vi "Log Events.vi"(2 "File Name":string, 3 "Log Path":path, 4 "Error In":errorcluster, 5 "Event":string, 6 "Time Format":string="%y/%m/%d; %H:%M:%S%3u", 7 "Log Command":T1) -> (0 "Error Out":errorcluster, 1 ">10MB":bool)   [LabVIEW 2018]
uses:
  Type Defs/Log Command.ctl
  <userlib>/_OpenG.lib/file/file.llb/Strip Path Extension - String__ogtk.vi
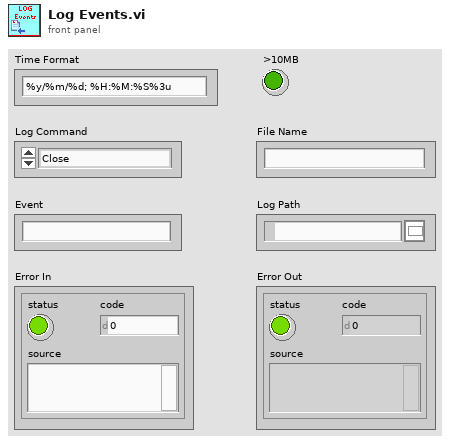
[diagram p1: front panel]
types:
  T1 = typedef "Log Command.ctl" = enum16{"Close", "Write", "Open", "No Command"}
  T2 = enum16{"open", "replace", "create", "open or create", "replace or create", "replace or create with confirmation"}
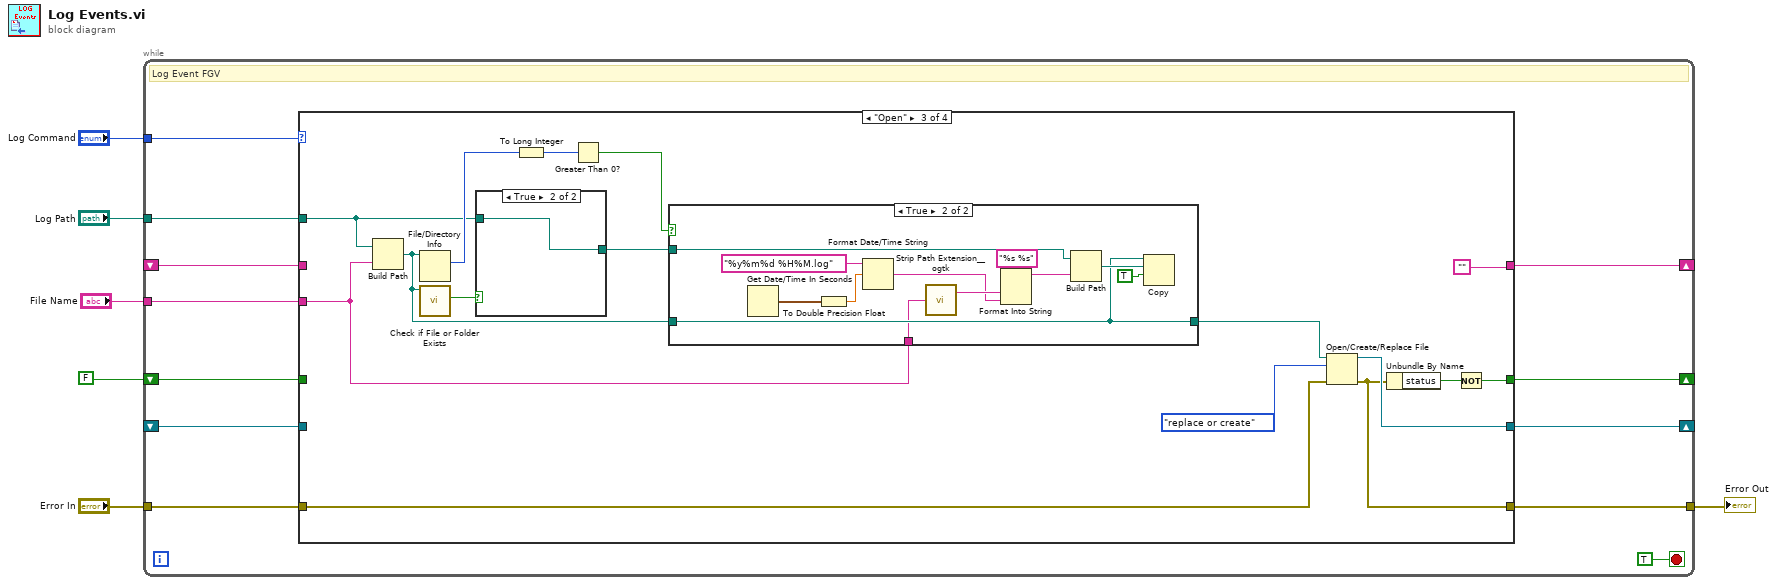
[diagram p0: block diagram]
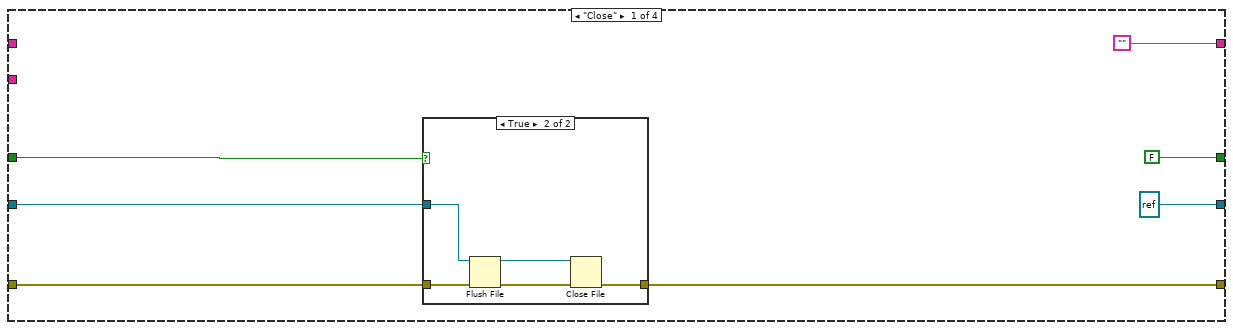
[diagram p2: hidden frame]
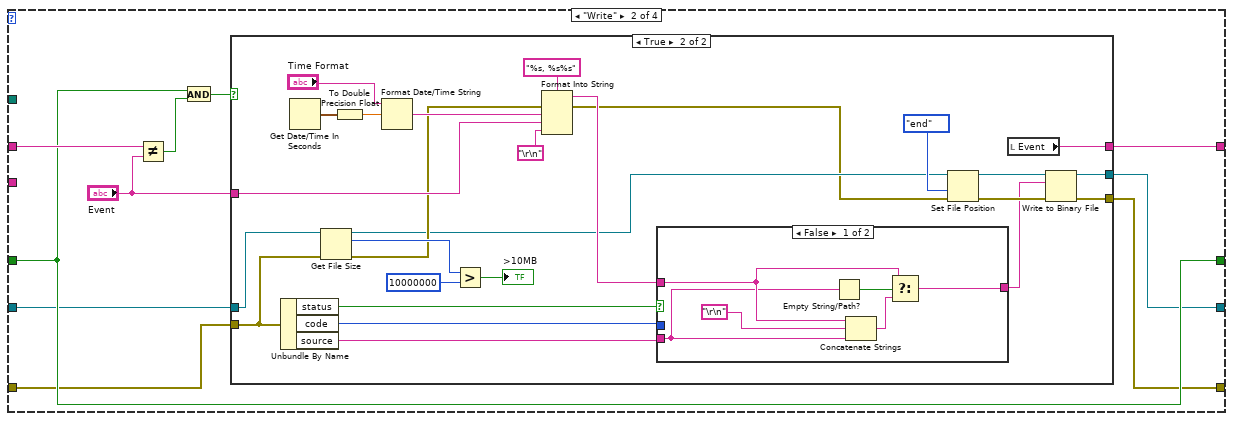
[diagram p4: hidden frame]
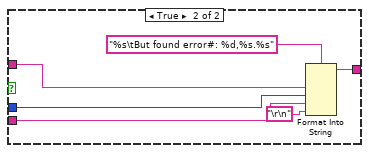
[diagram p6: hidden frame]
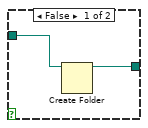
[diagram p7: hidden frame]
diagram:
  n1 = while {
    tunnel: "Error In" -> [w18]
    tunnel: [w17] -> w5
    tunnel: "Log Command" -> [w15]
    tunnel: "Log Path" -> [w14]
    tunnel: "File Name" -> [w13]
    shift-right: [w7] -> _
    shift-left: _ -> [w12]
    shift-right: [w10] -> _
    shift-left: FALSE -> [w11]
    shift-right: [w8] -> _
    shift-left: _ -> [w9]
    stop <- TRUE stop-if-true
    # "Log Event FGV"
    n2 = case shown="\"Open\"" w15 {
      tunnel: w18 -> [w24 w37 w86 w118]
      tunnel: [w22 w35 w87 w118] -> w17
      tunnel: w14 -> [_ _ w85 _]
      tunnel: w13 -> [_ _ w83 _]
      tunnel: w12 -> [w23 w34 _ w116]
      tunnel: w11 -> [w25 w39 _ w117]
      tunnel: [FALSE w39 w89 w117] -> w10
      tunnel: [refnum<file> refnum ("refnum out") w33 w88 w116] -> w7
      tunnel: w9 -> [_ w40 _ w115]
      tunnel: ["" w32 "" w115] -> w8
      frame "Close" {
        n3 = case shown="True" w25 {
          tunnel: w24 -> [w26 w28]
          tunnel: w23 -> [_ w29]
          tunnel: [w26 w27] -> w22
          frame False {
          }
          frame True {
            n4 = Flush File(refnum=w29, error in=w28) -> (refnum out=w30:refnum<file>, error out=w31:errorcluster)
            n5 = Close File(refnum=w30, error in=w31) -> (error out=w27:errorcluster)  [unwired: 1 out]
          }
        }
      }
      frame "Write" {
        n6 = Not Equal?(x=w40, y="Event") -> (x != y?=w41:bool)
        n7 = And(x=w39, y=w41) -> (x .and. y?=w38:bool)
        n8 = case shown="True" w38 {
          tunnel: w37 -> [w44 w56]
          tunnel: "Event" -> [w42 w65]
          tunnel: [w44 w49] -> w35
          tunnel: w34 -> [w43 w57]
          tunnel: [w43 w47] -> w33
          tunnel: [w42 w45] -> w32
          frame False {
          }
          frame True {
            n9 = Unbundle By Name(w56) -> ("status"=w64:bool, "code"=w63:i32, "source"=w62:string)
            n10 = Get Date/Time In Seconds() -> (seconds since 1Jan1904=w66:timestamp)
            n11 = Get File Size(file=w57, error in=w56) -> (refnum out=w50:refnum<file>, size (in bytes)=w59:i64, 0:w55:errorcluster)
            n12 = To Double Precision Float(number=w66) -> (double precision float=w70:dbl)
            n13 = Format Date/Time String(time format string (%c)="Time Format", seconds (now)=w70) -> (date/time string=w69:string)  [unwired: 1 out]
            n14 = Greater?(x=w59, y=i64 10000000) -> (0:→">10MB":bool)
            n15 = Format Into String(format string="%s, %s%s" ("Format String"), error in=w55, w69, w65, "\r\n") -> (resulting string=w61:string, error out=w48:errorcluster)  [unwired: 1 in]
            n16 = case shown="False" w64 {
              tunnel: w63 -> [_ w82]
              tunnel: w61 -> [w74 w81]
              tunnel: [w71 w79] -> w46
              tunnel: w62 -> [w72 w78]
              frame False {
                n17 = Empty String/Path?(string/path=w72) -> (empty?=w76:bool)
                n18 = Concatenate Strings(w74, "\r\n", w72) -> (w75:string)
                n19 = Select(t=w74, s=w76, f=w75) -> (s? t:f=w71:string)
              }
              frame True {
                n20 = Format Into String(format string="%s\tBut found error#: %d,%s.%s" ("Format String"), w81, w82, w78, "\r\n") -> (resulting string=w79:string)  [unwired: 2 in, 1 out]
              }
            }
            n21 = Set File Position(refnum=w50, from (0:start)=enum16{"start", "end", "current"}."end" ("pos mode (0:2)"), error in=w48) -> (refnum out=w52:refnum<file>, error out=w51:errorcluster)  [unwired: 1 out]
            n22 = local read "Event"() -> (w45:string)
            n23 = Write to Binary File(file (use dialog)=w52, data=w46, error in=w51) -> (refnum out=w47:refnum<file>, error out=w49:errorcluster)  [unwired: 1 in, 3 out]
          }
        }
      }
      frame "Open" {
        n24 = Build Path(base path=w85, name or relative path=w83) -> (appended path=w90:path)
        n25 = File/Directory Info(path=w90) -> (size=w96:i64)  [unwired: 1 in, 6 out]
        n26 = call <vilib>:"Check if File or Folder Exists.vi"("path"=w90) -> ("file or folder exists?"=w91:bool)  [unwired: 8 in, 2 out]
        n27 = case shown="True" w91 {
          tunnel: [w100 w101] -> w92
          tunnel: w85 -> [w99 w101]
          frame False {
            n28 = Create Folder(path (use dialog)=w99) -> (created path=w100:path)  [unwired: 2 in, 2 out]
          }
          frame True {
          }
        }
        n29 = To Long Integer(number=w96) -> (32bit integer=w97:i32)
        n30 = Greater Than 0?(x=w97) -> (x > 0?=w95:bool)
        n31 = case shown="True" w95 {
          tunnel: w90 -> [w102 w108]
          tunnel: w92 -> [_ w114]
          tunnel: [w102 w108] -> w94
          tunnel: w83 -> [_ w103]
          frame False {
          }
          frame True {
            n32 = Get Date/Time In Seconds() -> (seconds since 1Jan1904=w112:timestamp)
            n33 = To Double Precision Float(number=w112) -> (double precision float=w113:dbl)
            n34 = Format Date/Time String(time format string (%c)="%y%m%d %H%M.log", seconds (now)=w113) -> (date/time string=w104:string)  [unwired: 1 out]
            n35 = call-poly <userlib>:"Strip Path Extension__ogtk.vi"("path"=w103) -> ("root"=w106:string)  [unwired: 1 out]
            n36 = Format Into String(format string="%s %s", w106, w104) -> (resulting string=w105:string)  [unwired: 2 in, 1 out]
            n37 = Build Path(base path=w114, name or relative path=w105) -> (appended path=w110:path)
            n38 = Copy(9:TRUE ("overwrite (F)"), 10:w110, 11:w108) -> ()  [unwired: 1 in, 4 out]
          }
        }
        n39 = Open/Create/Replace File(file path (use dialog)=w94, error in=w86, operation (0:open)=T2."replace or create") -> (refnum out=w88:refnum<file>, error out=w87:errorcluster)  [unwired: 3 in, 1 out]
        n40 = Unbundle By Name(w87) -> ("status"=w98:bool)
        n41 = Not(x=w98) -> (.not. x?=w89:bool)
      }
      frame "No Command", Default {
      }
    }
  }
  "Error Out" <- w5
